vi "DemoConfig.vi"() -> ()   [LabVIEW 2010, in "MonitorServer.lvlib"]
uses:
  MonitorServer.lvlib
  SubVIs/ModBUS Driver/Private/MBDRV_Command List.ctl
  SubVIs/ModBUS Driver/Private/MBDRV_Command Data.ctl
  SubVIs/ModBUS Driver/Private/MBDRV_Action.ctl
  SubVIs/ModBUS Driver/Private/MBDRV_Response List.ctl
  SubVIs/ModBUS Driver/Private/MBDRV_Response.ctl
  Serial Config.ctl
panel:
  in  "Tab Control":T1(tab)
  in  "Start":bool
  in  "Stop":bool
  in  "Exit":bool
  in  "Config":bool
  in  "DeviceList":T2[](array[typedef])
  in  "Command":bool
  in  "Write To PLC":T3
  out "Read From PLC":T6
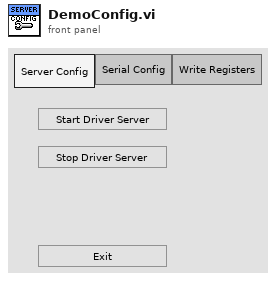
[diagram p1: front panel]
types:
  T1 = enum32{"Server Config", "Serial Config", "Write Registers"}
  T2 = typedef "MonitorServer.lvlib/Serial Config.ctl" = cluster{"设备名称":string, "串口选择":refnum<visa-resource-name>, "仪器地址":u32, "通讯速率":u32, "超时时间":u32, "刷新时间":dbl}
  T3 = typedef "MBDRV_Command List.ctl" = T4[]
  T4 = typedef "MBDRV_Command Data.ctl" = cluster{"Action":T5, "Com Port":string, "Register Address":u16, "Data To Write/Num To Read":i16}
  T5 = typedef "MBDRV_Action.ctl" = enum16{"Write", "Read"}
  T6 = typedef "MBDRV_Response List.ctl" = T7[]
  T7 = typedef "MBDRV_Response.ctl" = cluster{"Action":T5, "Com Port":string, "Register Address":u16, "Data":i16[]}
  T8 = enum32{"invalid app kind", "Development System", "Run Time System", "Student Edition", "Embedded LabVIEW", "Evaluation", "Custom"}
  T9 = enum32{"Invalid", "Standard", "Closed", "Hidden", "Minimized", "Maximized"}
  T10 = cluster{"Core":cluster{"Current VI Reference":refnum<vi>, "Close Panel on Exit?":bool}, "Your Boolean data":bool, "Your string data":string}
  T11 = cluster{"Current VI Reference":refnum<vi>, "Close Panel on Exit?":bool}
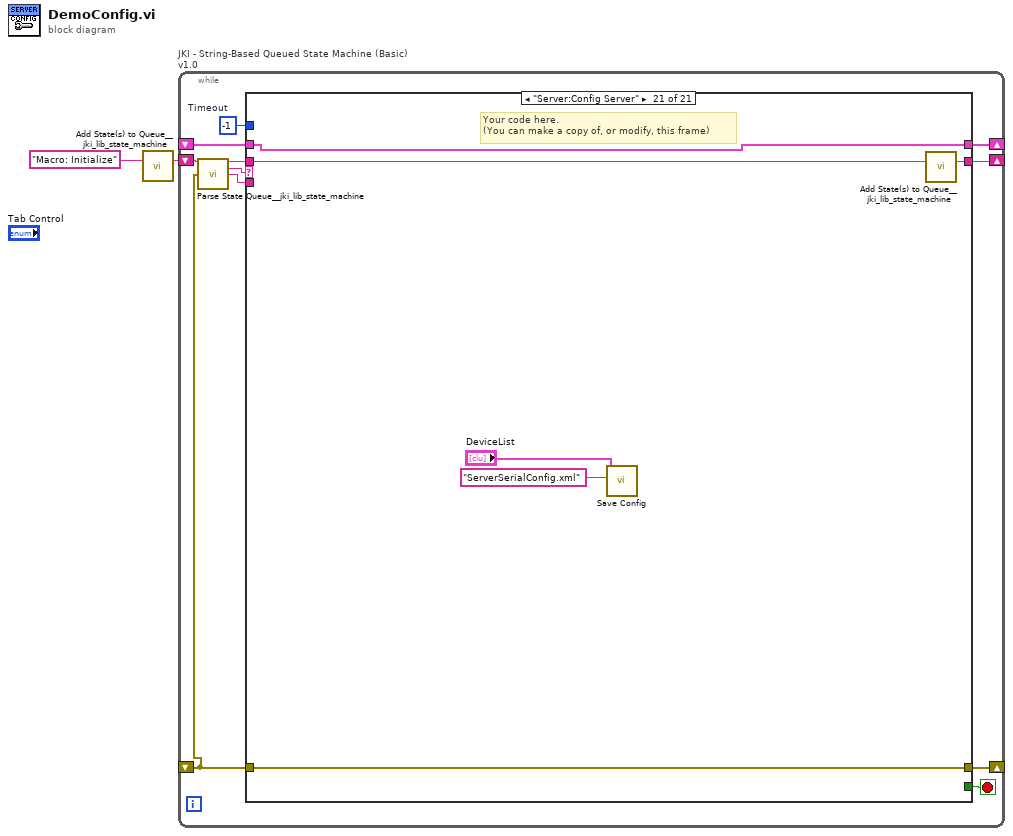
[diagram p0: block diagram]
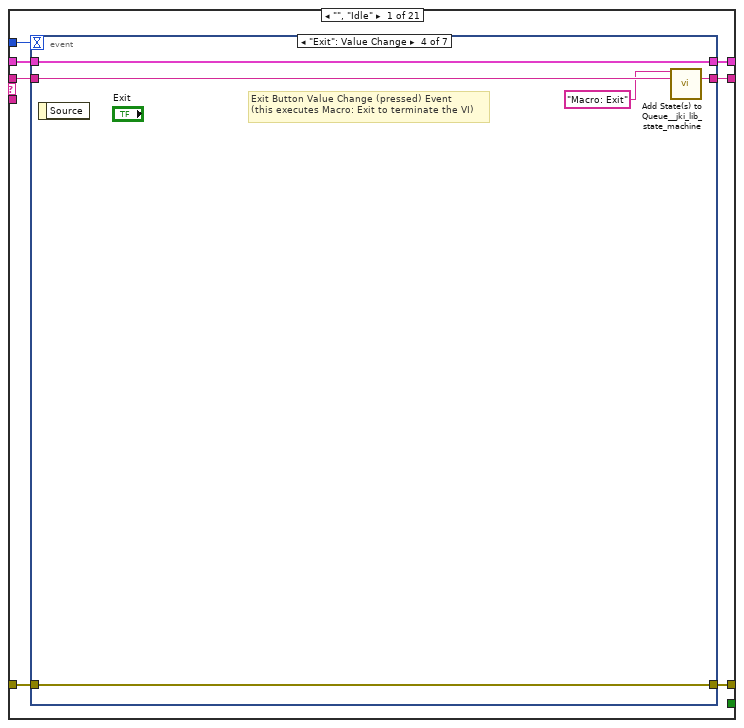
[diagram p2: hidden frame]
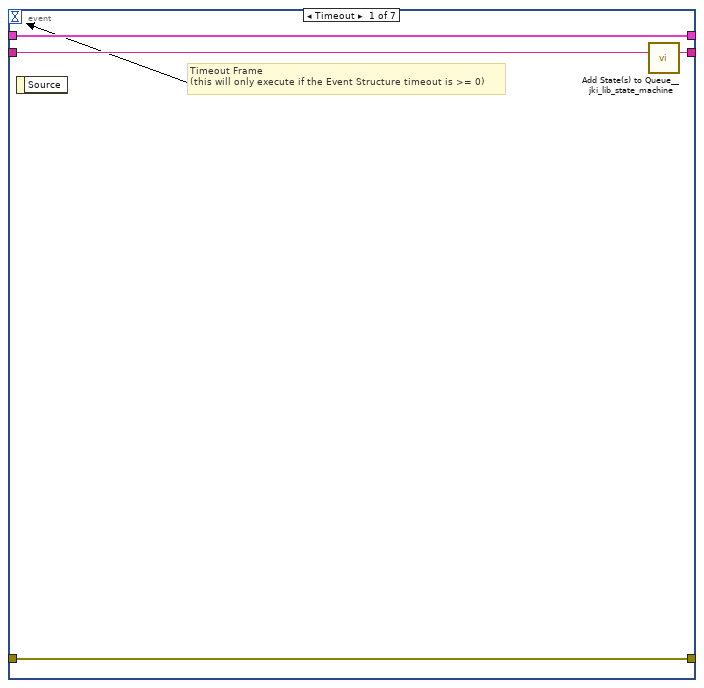
[diagram p3: hidden frame]
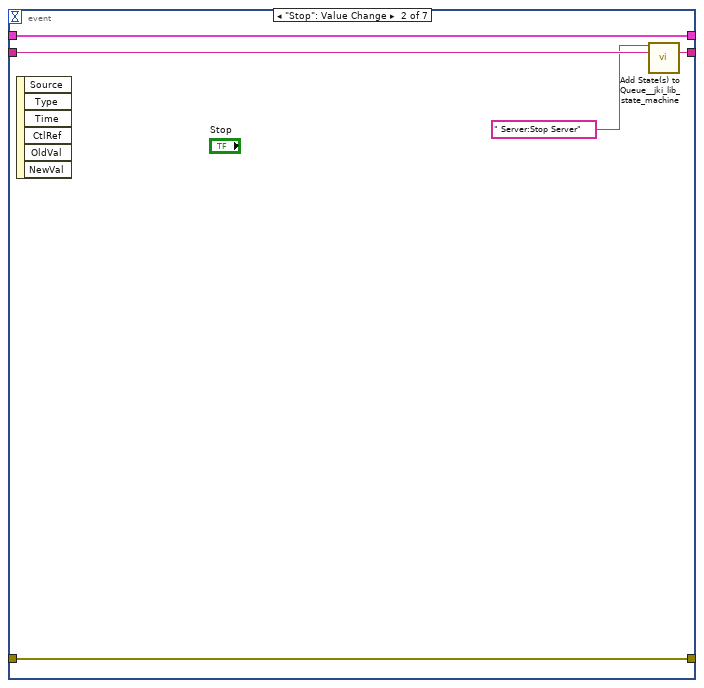
[diagram p4: hidden frame]
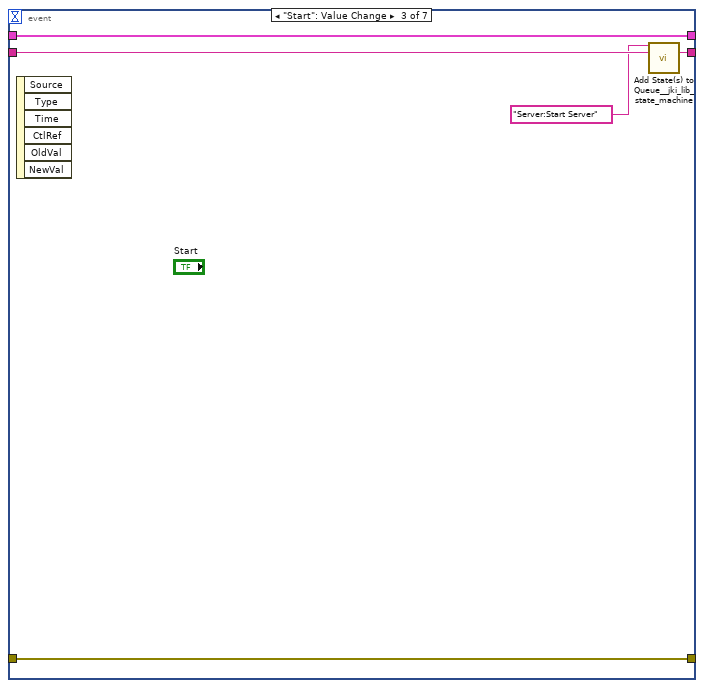
[diagram p5: hidden frame]
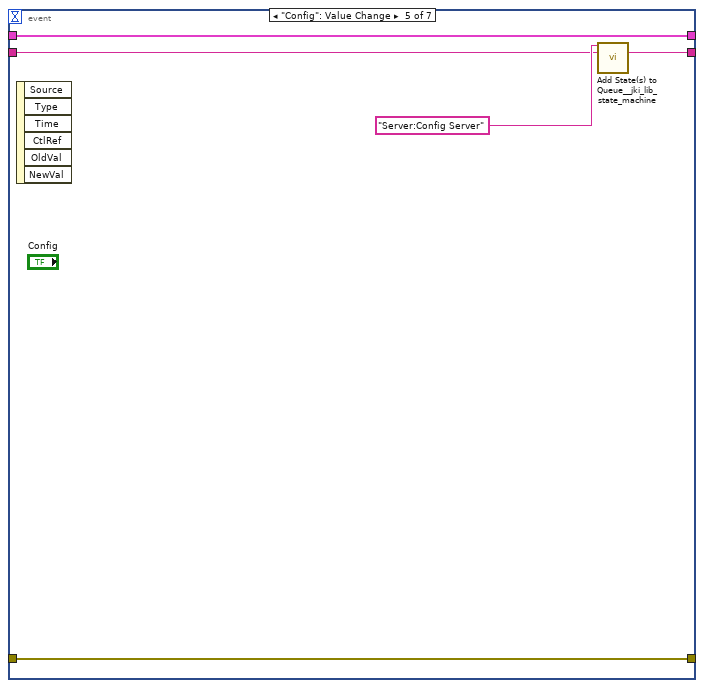
[diagram p6: hidden frame]
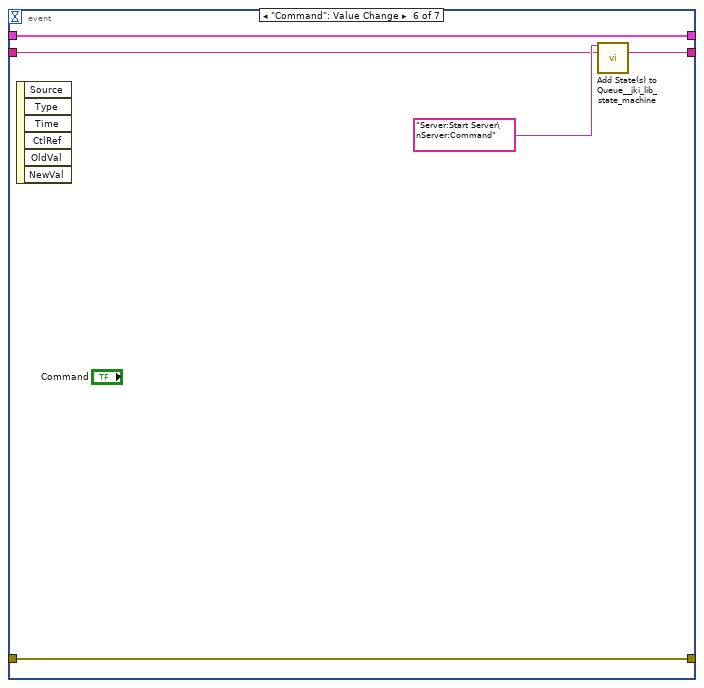
[diagram p7: hidden frame]
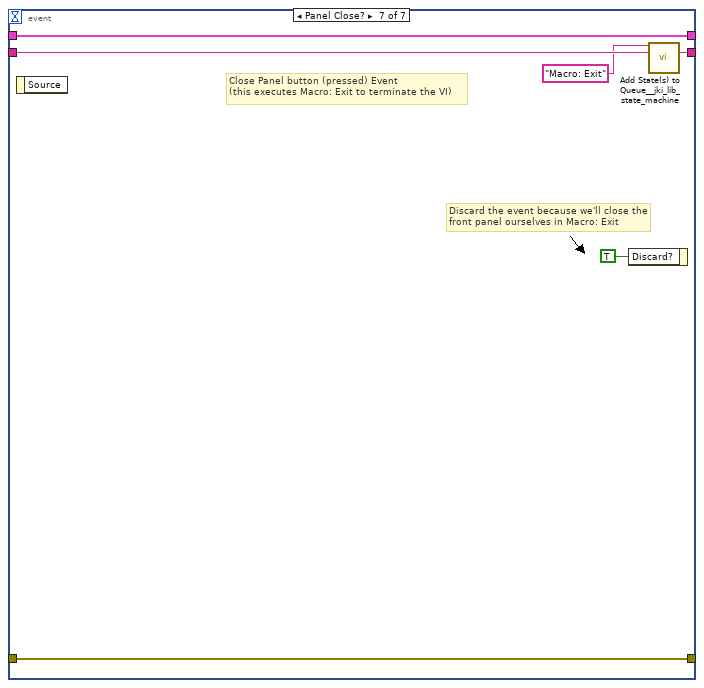
[diagram p8: hidden frame]
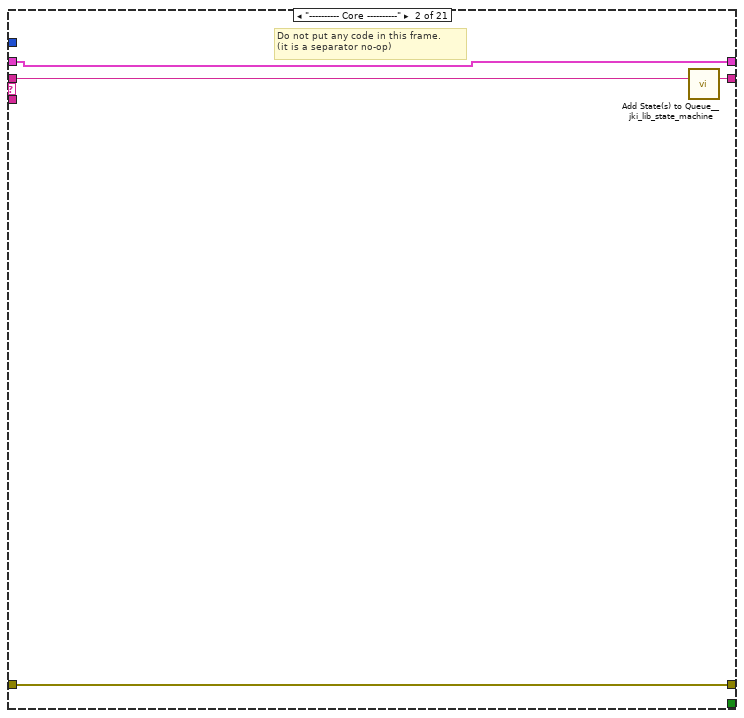
[diagram p9: hidden frame]
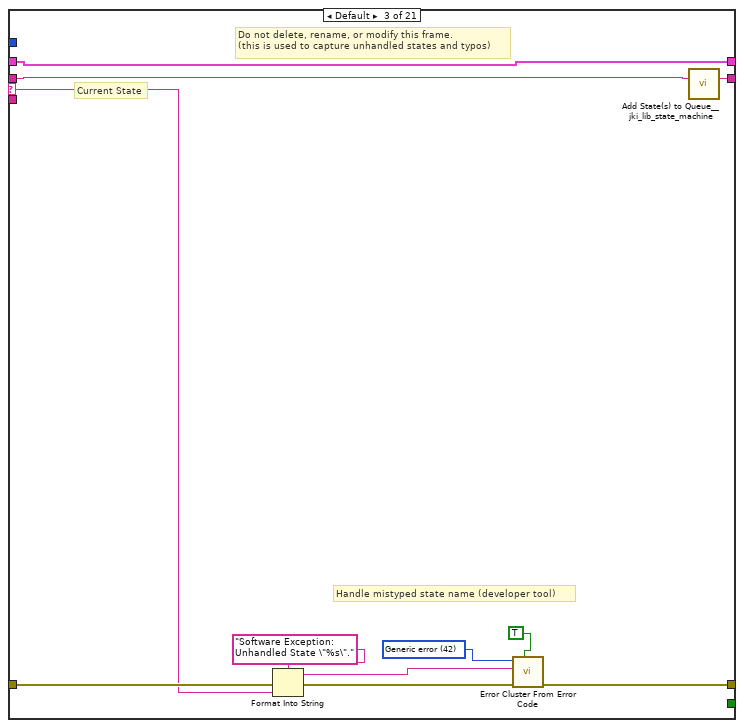
[diagram p10: hidden frame]
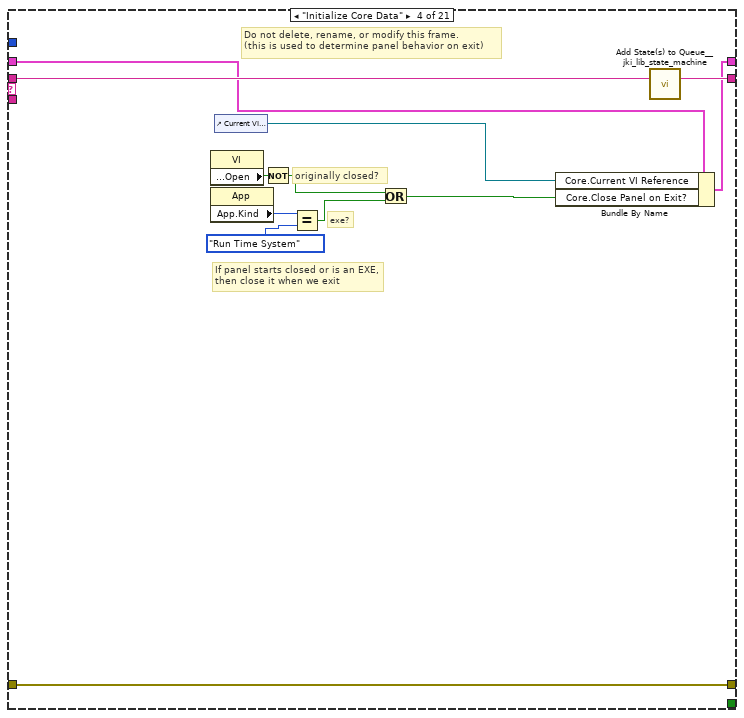
[diagram p11: hidden frame]
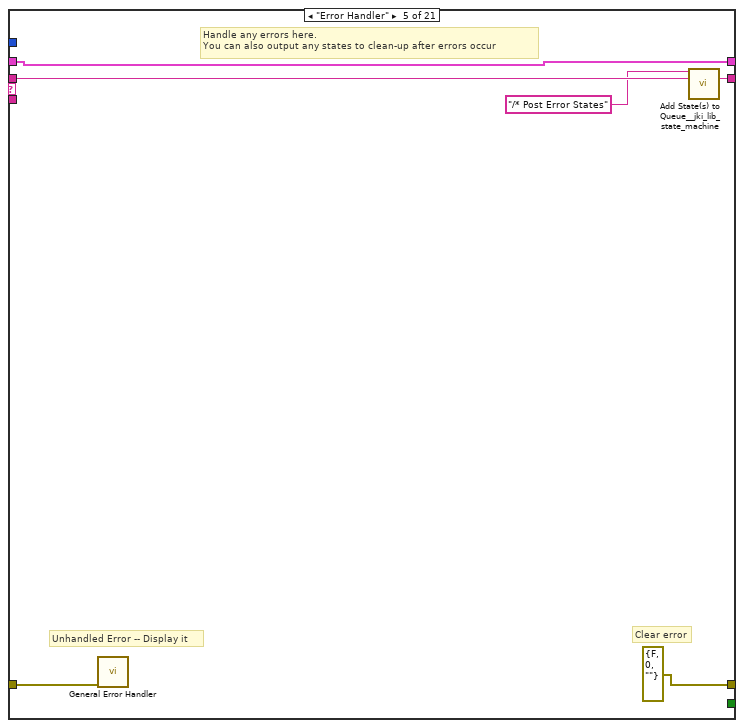
[diagram p12: hidden frame]
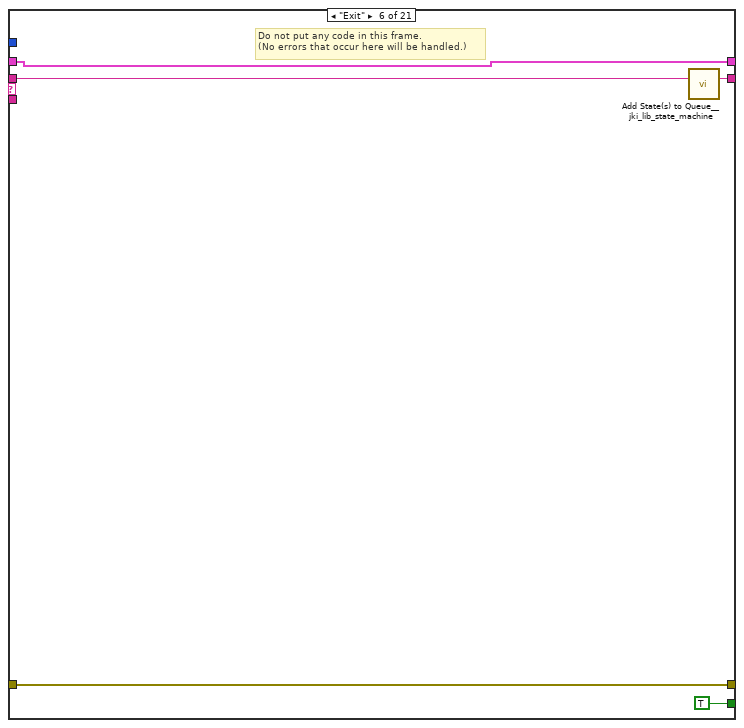
[diagram p13: hidden frame]
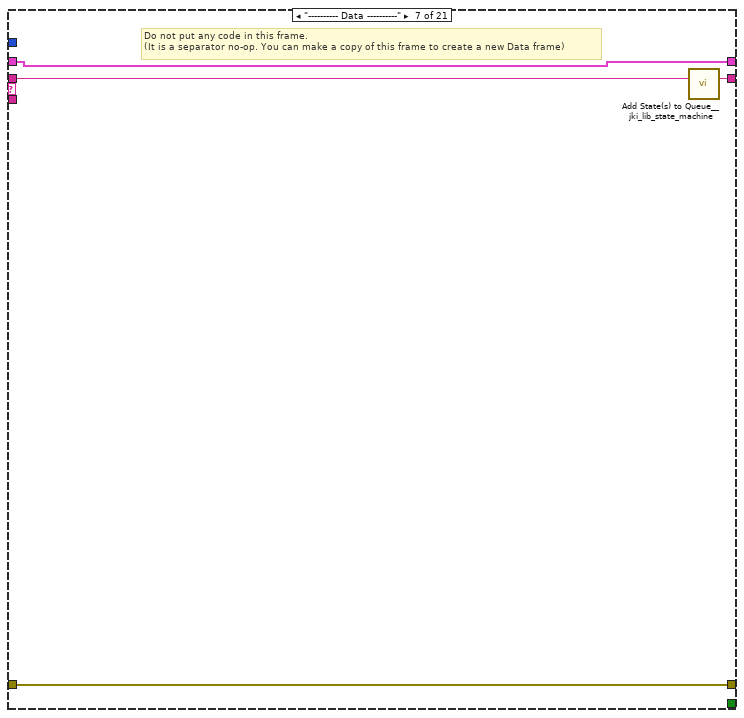
[diagram p14: hidden frame]
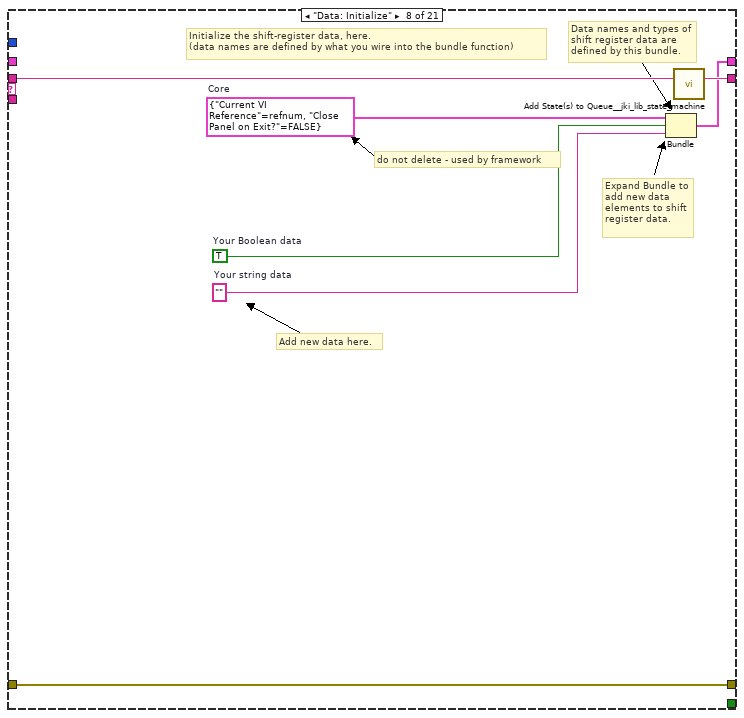
[diagram p15: hidden frame]
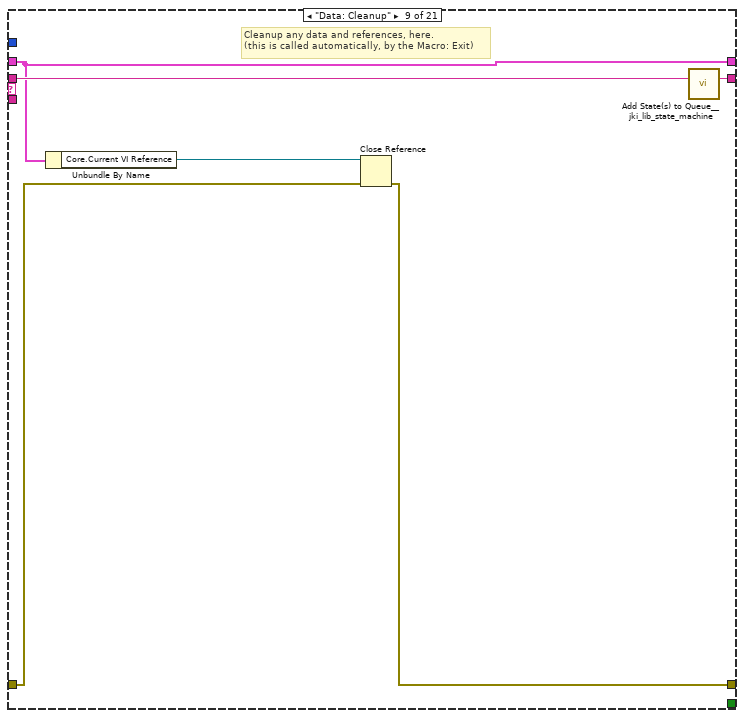
[diagram p16: hidden frame]
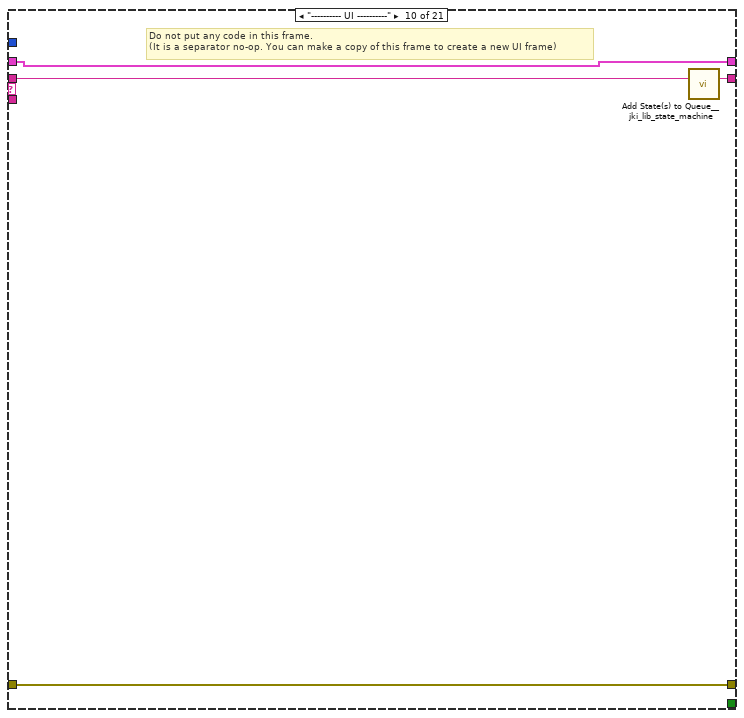
[diagram p17: hidden frame]
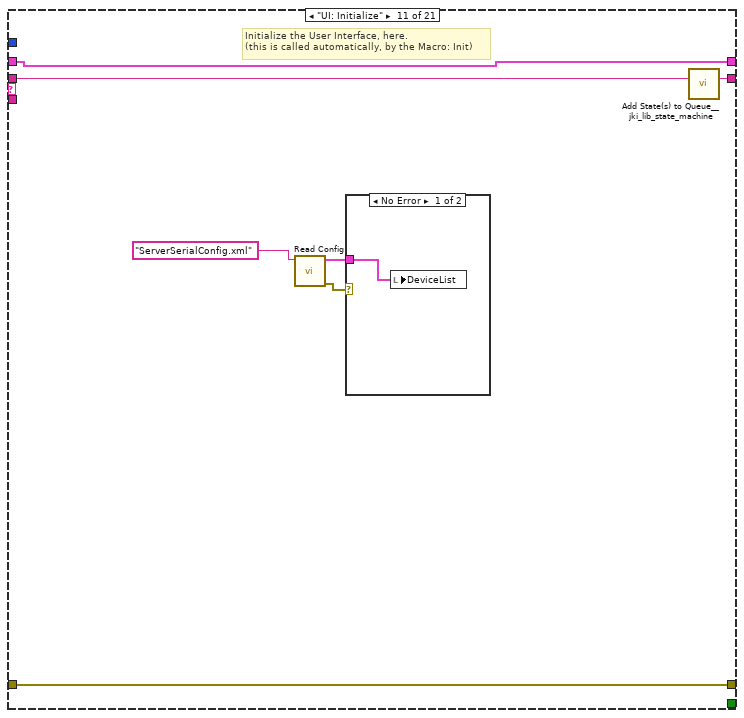
[diagram p18: hidden frame]
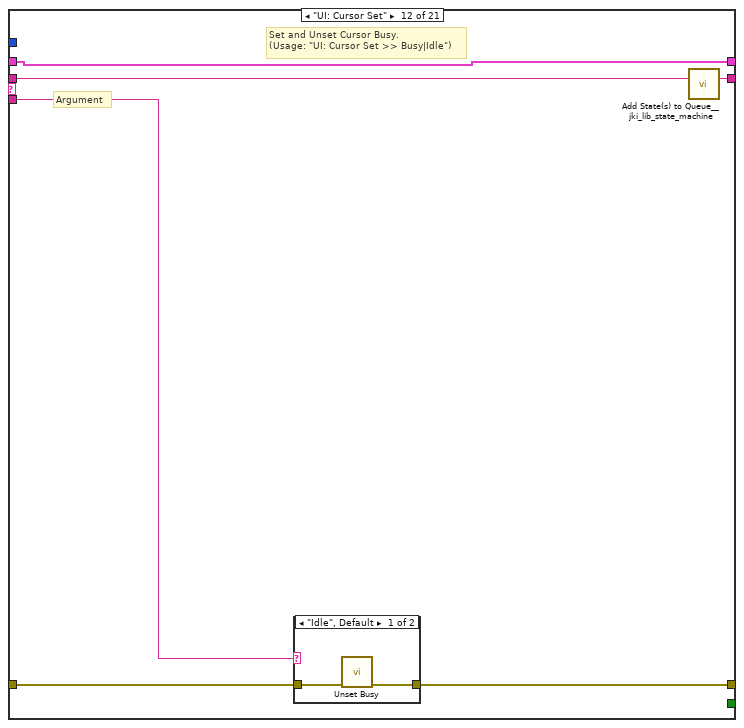
[diagram p20: hidden frame]
diagram:
  n1 = call "Add State(s) to Queue__jki_lib_state_machine.vi"("State(s) in (\"\")"="Macro: Initialize") -> ("States Out"=w2:string)  [unwired: 14 in]
  n2 = while "JKI - String-Based Queued State Machine (Basic) v1.0" {
    shift-right: [w6] -> _
    shift-left: _ -> [w5]
    shift-right: [w9] -> _
    shift-left: _ -> [w3]
    shift-right: [w8] -> _
    shift-left: w2 -> [w10]
    stop <- w7 stop-if-true
    w4 = -1  # Timeout
    n3 = call "Parse State Queue__jki_lib_state_machine.vi"("State Queue"=w10, "Error In (no error)"=w3) -> ("Remaining States"=w12:string, "Current State"=w13:string, "Arguments"=w11:string)  [unwired: 11 in]
    n4 = case shown="\"Server:Config Server\"" w13 {
      selector: w13 -> [_ _ w60 _ _ _ _ _ _ _ _ _ _ _ _ _ _ _ _ _ _]
      tunnel: w12 -> [w20 w59 w64 w82 w88 w93 w97 w104 w110 w114 w121 w128 w139 w165 w171 w182 w186 w190 w194 w198 w213]
      tunnel: w11 -> [_ _ _ _ _ _ _ _ _ _ _ w123 w133 _ _ _ _ _ _ _ _]
      tunnel: w5 -> [w18 w56 w62 w73 w85 w91 w94 _ w105 w111 w119 w126 w135 w162 w168 w179 w183 w187 w191 w195 w210]
      tunnel: [w17 w57 w66 w79 errorcluster {"status"=FALSE, "code"=0, "source"=""} ("error out") w90 w95 w101 w106 w112 w118 w124 w136 w163 w169 w180 w184 w188 w192 w196 w211] -> w9
      tunnel: w3 -> [w16 w57 w65 w79 w84 w90 w95 w101 w107 w112 w118 w125 w137 w163 w169 w180 w184 w188 w192 w196 w211]
      tunnel: [w19 w58 w63 w81 w87 w92 w96 w103 w109 w113 w120 w127 w138 w164 w170 w181 w185 w189 w193 w197 w212] -> w8
      tunnel: [_ _ _ _ _ TRUE _ _ _ _ _ _ _ _ _ _ _ _ _ _ _] -> w7
      tunnel: [w15 w56 w62 w80 w85 w91 w94 w102 w105 w111 w119 w126 w135 w162 w168 w179 w183 w187 w191 w195 w210] -> w6
      tunnel: w4 -> [w14 _ _ _ _ _ _ _ _ _ _ _ _ _ _ _ _ _ _ _ _]
      frame "", "Idle" {
        n5 = event shown="[3] \"Exit\": Value Change" {
          selector: _ -> [_ _ _ _ _ _ _]
          dyn-events: _ -> [_ _ _ _ _ _ _]
          timeout: w14 -> [_ _ _ _ _ _ _]
          tunnel: w20 -> [w24 w29 w34 w39 w41 w46 w55]
          tunnel: [w23 w28 w33 w38 w40 w45 w54] -> w19
          tunnel: w18 -> [w21 w26 w31 w36 w44 w49 w52]
          tunnel: [w22 w27 w32 w37 w43 w48 w53] -> w17
          tunnel: w16 -> [w22 w27 w32 w37 w43 w48 w53]
          tunnel: [w21 w26 w31 w36 w44 w49 w52] -> w15
          event Timeout {
            # "Timeout Frame\n(this will only execute if the Event Structure timeout is >= 0)"
            n6 = event-data() -> ()  [unwired: 1 in, 1 out]
            n7 = call "Add State(s) to Queue__jki_lib_state_machine.vi"("State(s) in (\"\")"=w24) -> ("States Out"=w23:string)  [unwired: 14 in]
          }
          event "Stop": Value Change {
            n8 = event-data() -> ()  [unwired: 1 in, 6 out]
            n9 = call "Add State(s) to Queue__jki_lib_state_machine.vi"("State(s) in Front (\"\")"=" Server:Stop Server" ("State(s) in Front (\"\")"), "State(s) in (\"\")"=w29) -> ("States Out"=w28:string)  [unwired: 13 in]
          }
          event "Start": Value Change {
            n10 = event-data() -> ()  [unwired: 1 in, 6 out]
            n11 = call "Add State(s) to Queue__jki_lib_state_machine.vi"("State(s) in Front (\"\")"="Server:Start Server" ("State(s) in Front (\"\")"), "State(s) in (\"\")"=w34) -> ("States Out"=w33:string)  [unwired: 13 in]
          }
          event "Exit": Value Change {
            # "Exit Button Value Change (pressed) Event\n(this executes Macro: Exit to terminate the VI)"
            n12 = event-data() -> ()  [unwired: 1 in, 1 out]
            n13 = call "Add State(s) to Queue__jki_lib_state_machine.vi"("State(s) in Front (\"\")"="Macro: Exit", "State(s) in (\"\")"=w39) -> ("States Out"=w38:string)  [unwired: 13 in]
          }
          event "Config": Value Change {
            n14 = event-data() -> ()  [unwired: 1 in, 6 out]
            n15 = call "Add State(s) to Queue__jki_lib_state_machine.vi"("State(s) in Front (\"\")"="Server:Config Server" ("State(s) in Front (\"\")"), "State(s) in (\"\")"=w41) -> ("States Out"=w40:string)  [unwired: 13 in]
          }
          event "Command": Value Change {
            n16 = event-data() -> ()  [unwired: 1 in, 6 out]
            n17 = call "Add State(s) to Queue__jki_lib_state_machine.vi"("State(s) in Front (\"\")"="Server:Start Server\nServer:Command" ("State(s) in Front (\"\")"), "State(s) in (\"\")"=w46) -> ("States Out"=w45:string)  [unwired: 13 in]
          }
          event Panel Close? {
            # "Discard the event because we'll close the front panel ourselves in Macro: Exit"
            # "Close Panel button (pressed) Event\n(this executes Macro: Exit to terminate the VI)"
            n18 = event-data() -> ()  [unwired: 1 in, 1 out]
            n19 = event-data("Discard?"=TRUE) -> ()  [unwired: 1 in, 1 out]
            n20 = call "Add State(s) to Queue__jki_lib_state_machine.vi"("State(s) in Front (\"\")"="Macro: Exit", "State(s) in (\"\")"=w55) -> ("States Out"=w54:string)  [unwired: 13 in]
          }
        }
      }
      frame "---------- Core ----------" {
        # "Do not put any code in this frame.\n(it is a separator no-op)"
        n21 = call "Add State(s) to Queue__jki_lib_state_machine.vi"("State(s) in (\"\")"=w59) -> ("States Out"=w58:string)  [unwired: 14 in]
      }
      frame Default {
        w69 = 42 items=["No error", "Argument error", "Memory is full", "Out of zone", "End of file", "File already open", "Generic file I/O error", "File not found", "File permission error", "Disk is full", "Duplicate path", "Too many files open", "System feature not enabled", "Resource file not found", "Cannot add resource", "Resource not found", "Image not found", "Image memory error", "Pen does not exist", "Config type invalid", "Config token not found", "Config parse error", "Config memory error", "Bad external code format", "Bad external code offset", "External code not present", "Null window", "Destroy window error", "Null menu", "Print aborted", "Bad print record", "Print driver error", "Windows error during printing", "Memory error during printing", "Print dialog error", "Generic print error", "Invalid device refnum", "Device not found", "Device parameter error", "Device unit error", "Cannot open device", "Device call aborted", "Generic error", "Cancelled by user", "Object ID too low", "Object ID too high", "Object not in heap", "Unknown heap", "Unknown object (invalid DefProc)", "Unknown object (DefProc not in table)", "Message out of range", "Invalid (null) method", "Unknown message", "Manager call not supported", "Bad address", "Network operation in progress", "Network operation timed out", "Connection is busy", "Network attribute not supported", "Network error", "Address in use", "System out of memory", "Connection aborted", "Connection refused", "Not connected", "Already connected", "Connection closed", "Initialization error (interapplication manager)", "Bad occurrence", "Wait on unbound occurrence handler", "Occurrence queue overflow", "Datalog type conflict", "Unused", "Unrecognized type (interapplication manager)", "Memory corrupt", "Failed to make temporary DLL", "Old CIN version", "Drag socket not found", "Failed to load drop-object", "Failed to register OLE object", "Failed to release OLE object", "Format specifier type mismatch", "Unknown format specifier", "Too few format specifiers", "Too many format specifiers", "Scan failed", "Newer CIN version", "Error converting to variant", "Runtime menu error", "Password tampered", "Variant attribute not found", "Incompatible variant data type", "Event data is not available", "Event Store is not present", "Occurrence is not found", "Event Queue is not created", "Event info is not available", "Refnum passed is NULL", "Error retrieving Class GUID", "Error retrieving CoClass GUID", "Error retrieving TypeLib GUID.", "Bad built application magic bytes.", "Specific driver is different from the specific driver associated with the Logical Name.", "There is no session opened to the class driver.", "Max Error", "MAX - Error with config objects", "MAX - Error loading configuration", "MAX - Group not supported"]
        # "Current State"
        # "Do not delete, rename, or modify this frame.\n(this is used to capture unhandled states and typos)"
        # "Handle mistyped state name (developer tool)"
        n22 = Format Into String(format string="Software Exception: Unhandled State \"%s\"." ("message"), error in=w65, w60) -> (resulting string=w68:string, error out=w67:errorcluster)  [unwired: 1 in]
        n23 = call <vilib>:"Error Cluster From Error Code.vi"("show call chain? (False)"=TRUE, "error in (no error)"=w67, "error message (\"\")"=w68, "error code (0)"=w69) -> ("error out"=w66:errorcluster)  [unwired: 5 in]
        n24 = call "Add State(s) to Queue__jki_lib_state_machine.vi"("State(s) in (\"\")"=w64) -> ("States Out"=w63:string)  [unwired: 14 in]
      }
      frame "Initialize Core Data" {
        # "Do not delete, rename, or modify this frame.\n(this is used to determine panel behavior on exit)"
        # "originally closed?"
        # "exe?"
        # "If panel starts closed or is an EXE, then close it when we exit"
        n25 = property class="VI"() -> ("Front Panel.Open"=w78:bool)  [unwired: 2 in, 2 out]
        n26 = property class="App"() -> ("App.Kind"=w77:T8)  [unwired: 2 in, 2 out]
        n27 = control-ref of="Current VI Reference"() -> (w71:refnum<vi>)
        n28 = Not(x=w78) -> (.not. x?=w75:bool)
        n29 = Equal?(x=w77, y=T8."Run Time System" ("Application:Kind")) -> (x = y?=w74:bool)
        n30 = Or(x=w75, y=w74) -> (x .or. y?=w72:bool)
        n31 = Bundle By Name(cluster=w73, "Core.Current VI Reference"=w71, "Core.Close Panel on Exit?"=w72) -> (w80:T10)
        n32 = call "Add State(s) to Queue__jki_lib_state_machine.vi"("State(s) in (\"\")"=w82) -> ("States Out"=w81:string)  [unwired: 14 in]
      }
      frame "Error Handler" {
        # "Unhandled Error -- Display it"
        # "Handle any errors here.\nYou can also output any states to clean-up after errors occur"
        # "Clear error"
        n33 = call <vilib>:"General Error Handler.vi"("error in (no error)"=w84) -> ()  [unwired: 10 in, 5 out]
        n34 = call "Add State(s) to Queue__jki_lib_state_machine.vi"("State(s) in Front (\"\")"="/* Post Error States", "State(s) in (\"\")"=w88) -> ("States Out"=w87:string)  [unwired: 13 in]
      }
      frame "Exit" {
        # "Do not put any code in this frame.\n(No errors that occur here will be handled.)"
        n35 = call "Add State(s) to Queue__jki_lib_state_machine.vi"("State(s) in (\"\")"=w93) -> ("States Out"=w92:string)  [unwired: 14 in]
      }
      frame "---------- Data ----------" {
        # "Do not put any code in this frame.\n(It is a separator no-op. You can make a copy of this frame to create a new Data frame)"
        n36 = call "Add State(s) to Queue__jki_lib_state_machine.vi"("State(s) in (\"\")"=w97) -> ("States Out"=w96:string)  [unwired: 14 in]
      }
      frame "Data: Initialize" {
        w98 = T11 {"Current VI Reference"=refnum, "Close Panel on Exit?"=FALSE}  # Core
        w100 = TRUE  # Your Boolean data
        w99 = ""  # Your string data
        # "do not delete - used by framework"
        # "Expand Bundle to add new data elements to shift register data."
        # "Add new data here."
        # "Data names and types of shift register data are defined by this bundle."
        # "Initialize the shift-register data, here.\n(data names are defined by what you wire into the bundle function)"
        n37 = Bundle("Core"=w98, "Your Boolean data"=w100, "Your string data"=w99) -> (w102:T10)  [unwired: 1 in]
        n38 = call "Add State(s) to Queue__jki_lib_state_machine.vi"("State(s) in (\"\")"=w104) -> ("States Out"=w103:string)  [unwired: 14 in]
      }
      frame "Data: Cleanup" {
        # "Cleanup any data and references, here.\n(this is called automatically, by the Macro: Exit)"
        n39 = Unbundle By Name(w105) -> ("Core.Current VI Reference"=w108:refnum<vi>)
        n40 = Close Reference(reference=w108, error in (no error)=w107) -> (error out=w106:errorcluster)
        n41 = call "Add State(s) to Queue__jki_lib_state_machine.vi"("State(s) in (\"\")"=w110) -> ("States Out"=w109:string)  [unwired: 14 in]
      }
      frame "---------- UI ----------" {
        # "Do not put any code in this frame.\n(It is a separator no-op. You can make a copy of this frame to create a new UI frame)"
        n42 = call "Add State(s) to Queue__jki_lib_state_machine.vi"("State(s) in (\"\")"=w114) -> ("States Out"=w113:string)  [unwired: 14 in]
      }
      frame "UI: Initialize" {
        # "Initialize the User Interface, here.\n(this is called automatically, by the Macro: Init)"
        n43 = call "Read Config.vi"("ConfigurationFileName"="ServerSerialConfig.xml" ("FileName")) -> ("error out"=w115:errorcluster, "DeviceList"=w116:T2[])  [unwired: 9 in]
        n44 = case shown="No Error" w115 {
          tunnel: w116 -> [w122 _]
          frame No Error {
            n45 = local write "DeviceList"(w122) -> ()
          }
          frame Error {
          }
        }
        n46 = call "Add State(s) to Queue__jki_lib_state_machine.vi"("State(s) in (\"\")"=w121) -> ("States Out"=w120:string)  [unwired: 14 in]
      }
      frame "UI: Cursor Set" {
        # "Argument"
        # "Set and Unset Cursor Busy.\n(Usage: \"UI: Cursor Set >> Busy|Idle\")"
        n47 = case shown="\"Idle\", Default" w123 {
          tunnel: w125 -> [w130 w132]
          tunnel: [w129 w131] -> w124
          frame "Idle", Default {
            n48 = call <vilib>:"Unset Busy.vi"("error in (no error)"=w130) -> ("error out"=w129:errorcluster)  [unwired: 10 in]
          }
          frame "Busy" {
            n49 = call <vilib>:"Set Busy.vi"("error in (no error)"=w132) -> ("error out"=w131:errorcluster)  [unwired: 9 in, 1 out]
          }
        }
        n50 = call "Add State(s) to Queue__jki_lib_state_machine.vi"("State(s) in (\"\")"=w128) -> ("States Out"=w127:string)  [unwired: 14 in]
      }
      frame "UI: Front Panel State" {
        # "Argument"
        # "Set Front Panel Open or Closed\n(Usage: \"UI: Front Panel State >> Open|Close\")"
        n51 = Unbundle By Name(w135) -> ("Core.Current VI Reference"=w134:refnum<vi>)
        n52 = case shown="\"Open\", Default" w133 {
          tunnel: w137 -> [w143 w156]
          tunnel: [w145 w157] -> w136
          tunnel: w134 -> [w144 w154]
          frame "Open", Default {
            n53 = property class="VI"(reference=w144, error in=w143) -> (reference out=w141:refnum<vi>, error out=w142:errorcluster, "Front Panel.Open"=w140:bool)
            n54 = case shown="True" w140 {
              tunnel: [w148 w151] -> w145
              tunnel: w142 -> [w147 w151]
              tunnel: w141 -> [w146 _]
              frame False {
                n55 = invoke class="VI" method="FP.Open"(reference=w146, error in=w147, "Activate"=TRUE, "State"=T9."Standard") -> (error out=w148:errorcluster)  [unwired: 1 in, 4 out]
              }
              frame True {
              }
            }
          }
          frame "Close" {
            n56 = property class="VI"(reference=w154, error in=w156) -> (reference out=w153:refnum<vi>, error out=w155:errorcluster, "Front Panel.Open"=w152:bool)
            n57 = case shown="True" w152 {
              tunnel: [w158 w161] -> w157
              tunnel: w155 -> [w158 w160]
              tunnel: w153 -> [_ w159]
              frame False {
              }
              frame True {
                n58 = invoke class="VI" method="FP.Close"(reference=w159, error in=w160) -> (error out=w161:errorcluster)  [unwired: 1 in, 2 out]
              }
            }
          }
        }
        n59 = call "Add State(s) to Queue__jki_lib_state_machine.vi"("State(s) in (\"\")"=w139) -> ("States Out"=w138:string)  [unwired: 14 in]
      }
      frame "---------- Macro ----------" {
        # "Do not put any code in this frame.\n(It is a separator no-op. You can make a copy of this frame to create a new Macro frame)"
        n60 = call "Add State(s) to Queue__jki_lib_state_machine.vi"("State(s) in (\"\")"=w165) -> ("States Out"=w164:string)  [unwired: 14 in]
      }
      frame "Macro: Initialize" {
        w167 = "Data: Initialize\nInitialize Core Data\nUI: Initialize\nUI: Front Panel State >> Open"  # Data: Initialize Initialize Core Data UI: Initialize UI: Front Panel State >> Open
        # "Initialization Macro\n(This is called once, when the VI starts)"
        n61 = shared-variable "My Computer\\MonitorServer.lvlib\\Server Status"("Working" ("Server Status")) -> ()  [unwired: 1 in, 1 out]
        n62 = call "Add State(s) to Queue__jki_lib_state_machine.vi"("State(s) in Front (\"\")"=w167, "State(s) in (\"\")"=w171) -> ("States Out"=w170:string)  [unwired: 13 in]
      }
      frame "Macro: Exit" {
        n63 = Unbundle By Name(w179) -> ("Core.Close Panel on Exit?"=w178:bool)
        n64 = shared-variable "My Computer\\MonitorServer.lvlib\\Server Status"("Stopped" ("Server Status")) -> ()  [unwired: 1 in, 1 out]
        n65 = Select(t="UI: Front Panel State >> Close", s=w178, f="") -> (s? t:f=w175:string)
        n66 = call "Add State(s) to Queue__jki_lib_state_machine.vi"("State(s) in (\"\")"=w175, "State(s) at Back (\"\")"="Data: Cleanup\nExit") -> ("States Out"=w173:string)  [unwired: 13 in]
        n67 = call "Add State(s) to Queue__jki_lib_state_machine.vi"("State(s) in Front (\"\")"=w173, "State(s) in (\"\")"=w182) -> ("States Out"=w181:string)  [unwired: 13 in]
      }
      frame "---------- Server ----------" {
        # "Template Separator\n(You can make a copy of, or modify, this frame)"
        n68 = call "Add State(s) to Queue__jki_lib_state_machine.vi"("State(s) in (\"\")"=w186) -> ("States Out"=w185:string)  [unwired: 14 in]
      }
      frame "Server:Start Server" {
        # "Your code here.\n(You can make a copy of, or modify, this frame)"
        n69 = call "StartServer.vi"() -> ()  [unwired: 11 in, 1 out]
        n70 = call "Add State(s) to Queue__jki_lib_state_machine.vi"("State(s) in (\"\")"=w190) -> ("States Out"=w189:string)  [unwired: 14 in]
      }
      frame "Server:Stop Server" {
        # "Your code here.\n(You can make a copy of, or modify, this frame)"
        n71 = call "StopServer.vi"() -> ()  [unwired: 11 in, 1 out]
        n72 = call "Add State(s) to Queue__jki_lib_state_machine.vi"("State(s) in (\"\")"=w194) -> ("States Out"=w193:string)  [unwired: 14 in]
      }
      frame "Server:Command" {
        # "Your code here.\n(You can make a copy of, or modify, this frame)"
        n73 = stacked-sequence {
          frame #0 {
            n74 = shared-variable "My Computer\\MonitorServer.lvlib\\Write To PLC"("Write To PLC") -> ()  [unwired: 1 in, 1 out]
          }
          frame #1 {
            n75 = shared-variable "My Computer\\MonitorServer.lvlib\\Command"("Register:Write" ("Command")) -> ()  [unwired: 1 in, 1 out]
          }
          frame #2 {
            n76 = for {
              N: 100 -> [_]
              stop <- w202 stop-if-true
              n77 = shared-variable "My Computer\\MonitorServer.lvlib\\Server Status"() -> (w205:string)  [unwired: 1 in, 1 out]
              n78 = Wait (ms)(milliseconds to wait=u32 100) -> ()  [unwired: 1 out]
              n79 = Equal?(x=w205, y="Finish") -> (x = y?=w202:bool)
            }
          }
          frame #3 {
            n80 = shared-variable "My Computer\\MonitorServer.lvlib\\Read From PLC"() -> (→"Read From PLC":T6)  [unwired: 1 in, 1 out]
            n81 = shared-variable "My Computer\\MonitorServer.lvlib\\Server Status"("" ("Server Status")) -> ()  [unwired: 1 in, 1 out]
          }
        }
        n82 = call "Add State(s) to Queue__jki_lib_state_machine.vi"("State(s) in (\"\")"=w198) -> ("States Out"=w197:string)  [unwired: 14 in]
      }
      frame "Server:Config Server" {
        # "Your code here.\n(You can make a copy of, or modify, this frame)"
        n83 = call "Save Config.vi"("FileName"="ServerSerialConfig.xml", "DeviceList"="DeviceList") -> ()  [unwired: 9 in, 1 out]
        n84 = call "Add State(s) to Queue__jki_lib_state_machine.vi"("State(s) in (\"\")"=w213) -> ("States Out"=w212:string)  [unwired: 14 in]
      }
    }
  }
